vi "LIA_7230_Messgearet.vi"(1 "refnum":refnum<file>, 2 "Numerisch":i8 min=0 max=2 step=1) -> ()   [LabVIEW 2019]
uses:
  Global/Global Variables/Data_Display_global.vi
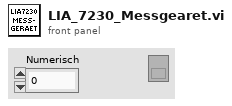
[diagram p1: front panel]
types:
  T1 = typedef "LIA7230-cluster.ctl" = cluster{"Lockin 1":dbl[][], "X1-Display":dbl, "X1 Percent":dbl, "Y1-Display":dbl, "X1 Percent 2":dbl, "Unit X1":string, "Unit X2":string, "X1 Overload":bool, "Y1 Overload":bool, "Sensitivity Setpoint":i16, "X1":dbl, "Y1":dbl, "Channel 3":dbl, "Channel 4":dbl, "Channel 4 Percent":dbl, "Channel 3 Percent ":dbl, "Unit Channel 3":string, "Unit Channel 4":string, "Overload channel 3":bool, "Overload channel 4":bool, "Offsets (ON)":bool, "Sensitivity Setpoint 2":i16}
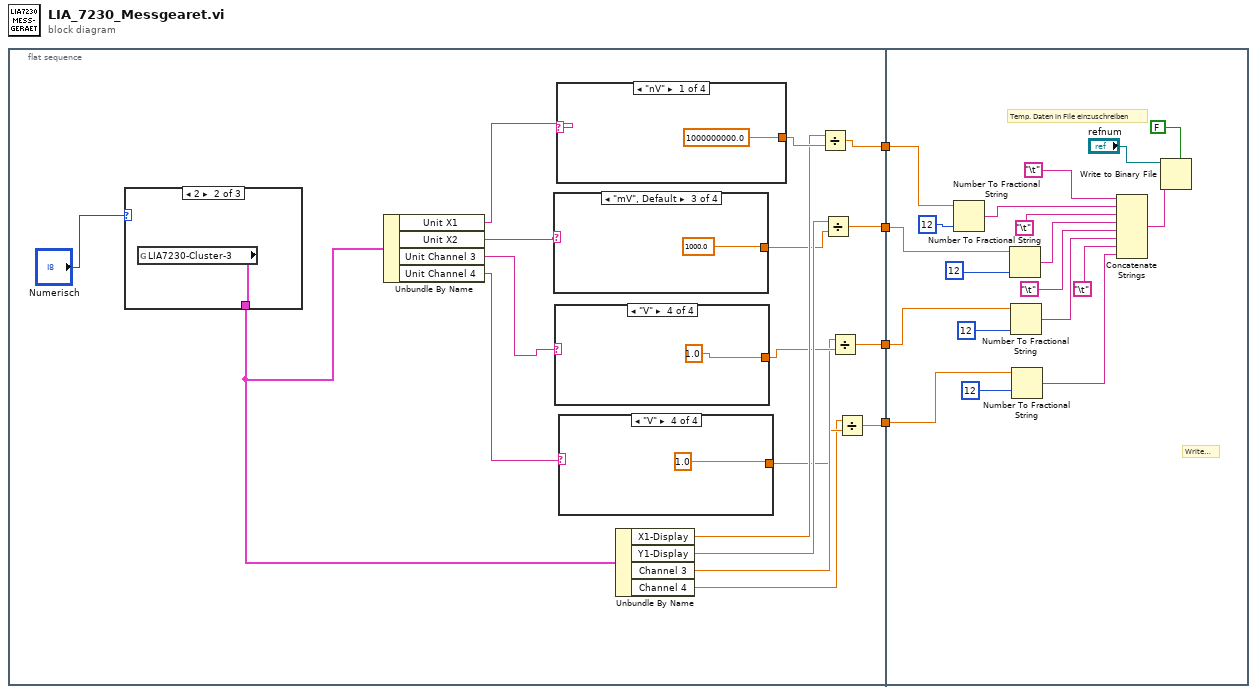
[diagram p0: block diagram]
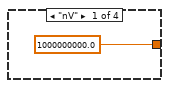
[diagram p2: hidden frame]
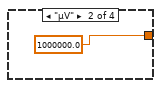
[diagram p3: hidden frame]
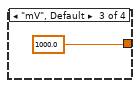
[diagram p4: hidden frame]
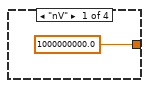
[diagram p5: hidden frame]
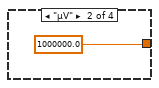
[diagram p6: hidden frame]
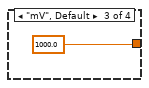
[diagram p7: hidden frame]
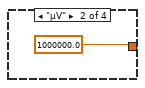
[diagram p8: hidden frame]
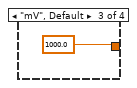
[diagram p9: hidden frame]
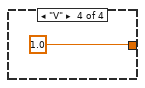
[diagram p10: hidden frame]
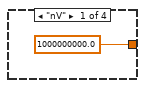
[diagram p11: hidden frame]
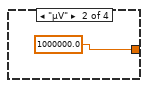
[diagram p12: hidden frame]
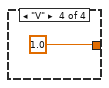
[diagram p13: hidden frame]
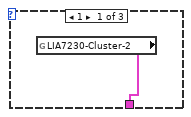
[diagram p14: hidden frame]
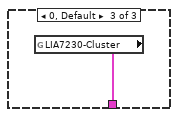
[diagram p15: hidden frame]
diagram:
  n1 = flat-sequence {
    tunnel: [w14] -> w4
    tunnel: [w11] -> w3
    tunnel: [w8] -> w2
    tunnel: [w5] -> w1
    tunnel: w4 -> [w51]
    tunnel: w3 -> [w50]
    tunnel: w2 -> [w49]
    tunnel: w1 -> [w43]
    frame #0 {
      n2 = case shown="2" "Numerisch" {
        tunnel: [w39 w40 w41] -> w22
        frame 1 {
          n3 = global read "Data_Display_global.vi" "LIA7230-Cluster-2"() -> (w39:T1)
        }
        frame 2 {
          n4 = global read "Data_Display_global.vi" "LIA7230-Cluster-3"() -> (w40:T1)
        }
        frame 0, Default {
          n5 = global read "Data_Display_global.vi" "LIA7230-Cluster"() -> (w41:T1)
        }
      }
      n6 = Unbundle By Name(w22) -> ("Unit X1"=w19:string, "Unit X2"=w20:string, "Unit Channel 3"=w18:string, "Unit Channel 4"=w17:string)
      n7 = case shown="\"mV\", Default" w20 {
        tunnel: [1000000000.0 1000000.0 1000.0 1.0] -> w12
        frame "nV" {
        }
        frame "µV" {
        }
        frame "mV", Default {
        }
        frame "V" {
        }
      }
      n8 = case shown="\"V\"" w18 {
        tunnel: [1000000000.0 1000000.0 1000.0 1.0] -> w10
        frame "nV" {
        }
        frame "µV" {
        }
        frame "mV", Default {
        }
        frame "V" {
        }
      }
      n9 = case shown="\"nV\"" w19 {
        tunnel: [1000000000.0 1000000.0 1000.0 1.0] -> w16
        frame "nV" {
        }
        frame "µV" {
        }
        frame "mV", Default {
        }
        frame "V" {
        }
      }
      n10 = case shown="\"V\"" w17 {
        tunnel: [1000000000.0 1000000.0 1000.0 1.0] -> w7
        frame "nV" {
        }
        frame "µV" {
        }
        frame "mV", Default {
        }
        frame "V" {
        }
      }
      n11 = Unbundle By Name(w22) -> ("X1-Display"=w15:dbl, "Y1-Display"=w13:dbl, "Channel 3"=w9:dbl, "Channel 4"=w6:dbl)
      n12 = Divide(x=w15, y=w16) -> (x/y=w14:dbl)
      n13 = Divide(x=w13, y=w12) -> (x/y=w11:dbl)
      n14 = Divide(x=w9, y=w10) -> (x/y=w8:dbl)
      n15 = Divide(x=w6, y=w7) -> (x/y=w5:dbl)
    }
    frame #1 {
      # "Temp. Daten in File einzuschreiben"
      # "Write File"
      n16 = Number To Fractional String(number=w51, precision (6)=i16 12) -> (F-format string=w58:string)  [unwired: 2 in]
      n17 = Number To Fractional String(number=w50, precision (6)=i16 12) -> (F-format string=w57:string)  [unwired: 2 in]
      n18 = Number To Fractional String(number=w49, precision (6)=12) -> (F-format string=w46:string)  [unwired: 2 in]
      n19 = Number To Fractional String(number=w43, precision (6)=12) -> (F-format string=w44:string)  [unwired: 2 in]
      n20 = Concatenate Strings("\t", w58, "\t", w57, "\t", w46, "\t", w44) -> (w60:string)
      n21 = Write to Binary File ("Write File")(file (use dialog)="refnum", data=w60, 5:FALSE ("prepend array or string size? (T)")) -> ()  [unwired: 3 in, 3 out]
    }
  }
